vi "Dashboard Main.vi"() -> ()   [LabVIEW 2016]
uses:
  <vilib>/Utility/miscctls.llb/LVRectTypeDef.ctl
  <vilib>/Utility/miscctls.llb/LVPointTypeDef.ctl
  System.Speech
  <vilib>/Rock Robotics/Network Tables/NT Write Number.vi
  <vilib>/Rock Robotics/Network Tables/NT Write Boolean.vi
  <vilib>/Rock Robotics/Network Tables/NT Read Number.vi
  <vilib>/Rock Robotics/Network Tables/NT Read Boolean.vi
  <vilib>/sound2/lvsound2.llb/Sound Output Write (DBL).vi
  Downloads/Beachbot2016Dash-master (1)/Beachbot2016Dash-master/Custom/BB_AutonomousSelector.lvlib
  <vilib>/vision/NI_Vision_Development_Module.lvlib
panel:
  out "Mask 2":T1(plugin-control)
  out "Mask":T1(plugin-control)
  out "Camera Image 2":T1(plugin-control)
  in  "TCP":refnum<k5>
  out "Robot IP":string
  in  "Dashboard Tab":T2(tab)
  out "Gear":u32(colorbox)
  out "NT Connection":bool
  out "Mode":T3(ring)=enum."Auto Disabled"
  out "Shooter RPM":dbl(knob) scale=0.0..3400.0
  out "Air Pressure":dbl(knob) scale=0.0..130.0
  out "Boiler Angle":dbl
  out "Boiler Distance":dbl
  out "In Range":bool=TRUE
  in  "Oscillate":bool=TRUE
  in  "Auto Program":u16(ring) items=["Right Boiler -R- Gear & Shoot", "Right Boiler -L- Gear & Hopper", "Right Boiler 40 Ball v2", "Right Boiler -C- Gear, Shoot & CATCH", "Left Boiler 40 Ball", "Do Nothing", "Right Boiler -C- Gear & Shoot", "Right Boiler -R- Gear Vision & Shoot", "Right Boiler -L- Gear & CATCH", "Left Boiler -C- Gear & Shoot", "Right Boiler 40 Ball", "Left Boiler -L- Gear & Shoot", "Right Boiler -L- Gear & SPRINT"]
  in  "AutoDelay":dbl
  out "MatchTime":i32
  in  "Airship Cam":bool
  in  "Driver Cam":bool
  in  "Shooter Cam":T4={"Hue"={126.19617640889274, 181.21165574429517}, "Sat"={179.10714285714286, 255.0}, "Val"={75.89285714285715, 179.10714285714286}} {"Hue" scale=0.0..255.0 scale format="%#_3g"}
  in  "Driver Cam":T4={"Hue"={104.14999988007006, 130.81818389892578}, "Sat"={157.85714285714286, 255.0}, "Val"={40.53571428571429, 212.5}} {"Hue" scale=0.0..255.0 scale format="%#_3g"}
  out "Tree":string(tree)
  out "Camera Image":T1(plugin-control)
  out "Background":bool
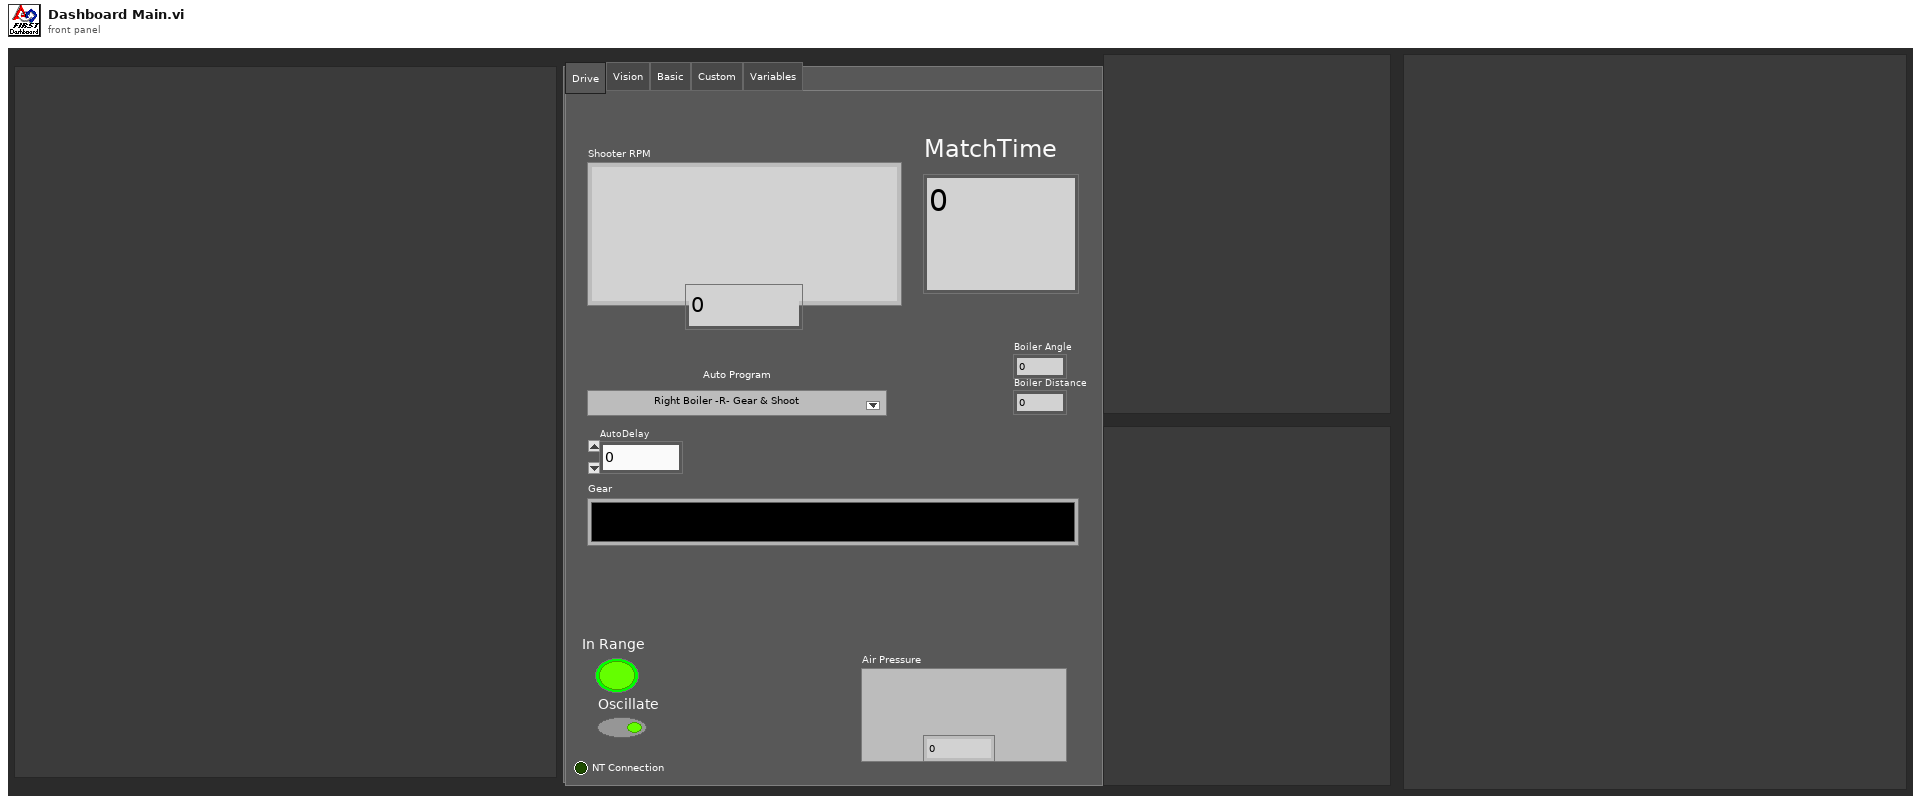
[diagram p1: front panel]
types:
  T1 = typedef "IMAQ Image.ctl" = refnum<image>
  T2 = enum32{"Drive", "Vision", "Basic", "Custom", "Variables"}
  T3 = enum8{"Tele-Op Disabled", "Tele-Op Enabled", "Auto Disabled", "Auto Enabled", "Test Disabled", "Test Enabled", "Disconnected", "No Code", "E-Stop"}
  T4 = cluster{"Hue":cluster{dbl, dbl}, "Sat":cluster{dbl, dbl}, "Val":cluster{dbl, dbl}}
  T5 = typedef "Image Type" = u32
  T6 = typedef "LVPointTypeDef.ctl" = cluster{"Horizontal":i16, "Vertical":i16}
  T7 = typedef "LVRectTypeDef.ctl" = cluster{"Left":i16, "Top":i16, "Right":i16, "Bottom":i16}
  T8 = enum32{"Drive", "Basic", "Custom", "Test", "Checklist", "Variables"}
  T9 = cluster{"Shift":bool, "Ctrl":bool, "Alt":bool, "Cmd":bool, "Opt":bool}
  T10 = cluster{"Error Strings":string, "Disable Counts":cluster{u16, u16}, "Rail Faults":cluster{u16, u16, u16}, "Robot IP":string, "DB Mode":u8, "Event Info":cluster{"Name":string, "Type":u8, "Number":u16, "Replay":u8}}
  T11 = cluster{"Storage":cluster{"Disk Free":u64, "RAM Block":u32, "RAM free":u32}, "CPU Utilization":cluster{"CPU % ISR":sgl, "CPU % Time Crit":sgl, "CPU % Timed Str":sgl, "CPU % High":sgl, "CPU % Above":sgl, "CPU % Normal":sgl, "CPU % Low":sgl}, "CAN":cluster{"% Bus Utilization":sgl, "Bus Off Cnt":u32, "TX_FIFO Full Cnt":u32, "Receive Error Cnt":u8, "Transmit Error Cnt":u8}, "HID":cluster{"HID Outputs":u32, "Rumble Low":u16, "Rumble High":u16}[]}
  T12 = cluster{"Status bits":cluster{"Test Mode":bool, "Autonomous":bool, "Enabled":bool, "Code Start":bool, "Brownout":bool, "Reserved 2":bool, "Reserved 3":bool, "E-Stop":bool}, "Code Trace":cluster{"Disabled":bool, "TeleOp":bool, "Auto":bool, "Test":bool}, "Controller Type":enum16{"unknown", "cRIO", "roboRio"}, "Code?":enum16{"unknown", "noCode", "code"}, "Battery V":dbl}
  T13 = cluster{"Control Bits":cluster{"TestMode":bool, "Autonomous":bool, "Enabled":bool, "FMS Present":bool, bool, bool, bool, "E-Stop":bool}, "Team Station ":u8, "Countdown":sgl, "Joystick Values":cluster{"Axes":dbl[], "Buttons":bool[], "POVs":i16[]}[]}
  T14 = typedef "Sound Output Task ID.ctl" = u32
  T15 = cluster{"Distance (ft)":dbl, "Score":dbl, "Normalized":cluster{"Center":cluster{dbl, dbl}, "Rectangle":cluster{"Numeric":dbl, "Numeric 2":dbl, "Numeric 3":dbl, "Numeric 5":dbl}}, "Pixels":cluster{"Center":cluster{dbl, dbl}, "Rectangle":cluster{"Numeric":dbl, "Numeric 2":dbl, "Numeric 3":dbl, "Numeric 5":dbl}}}
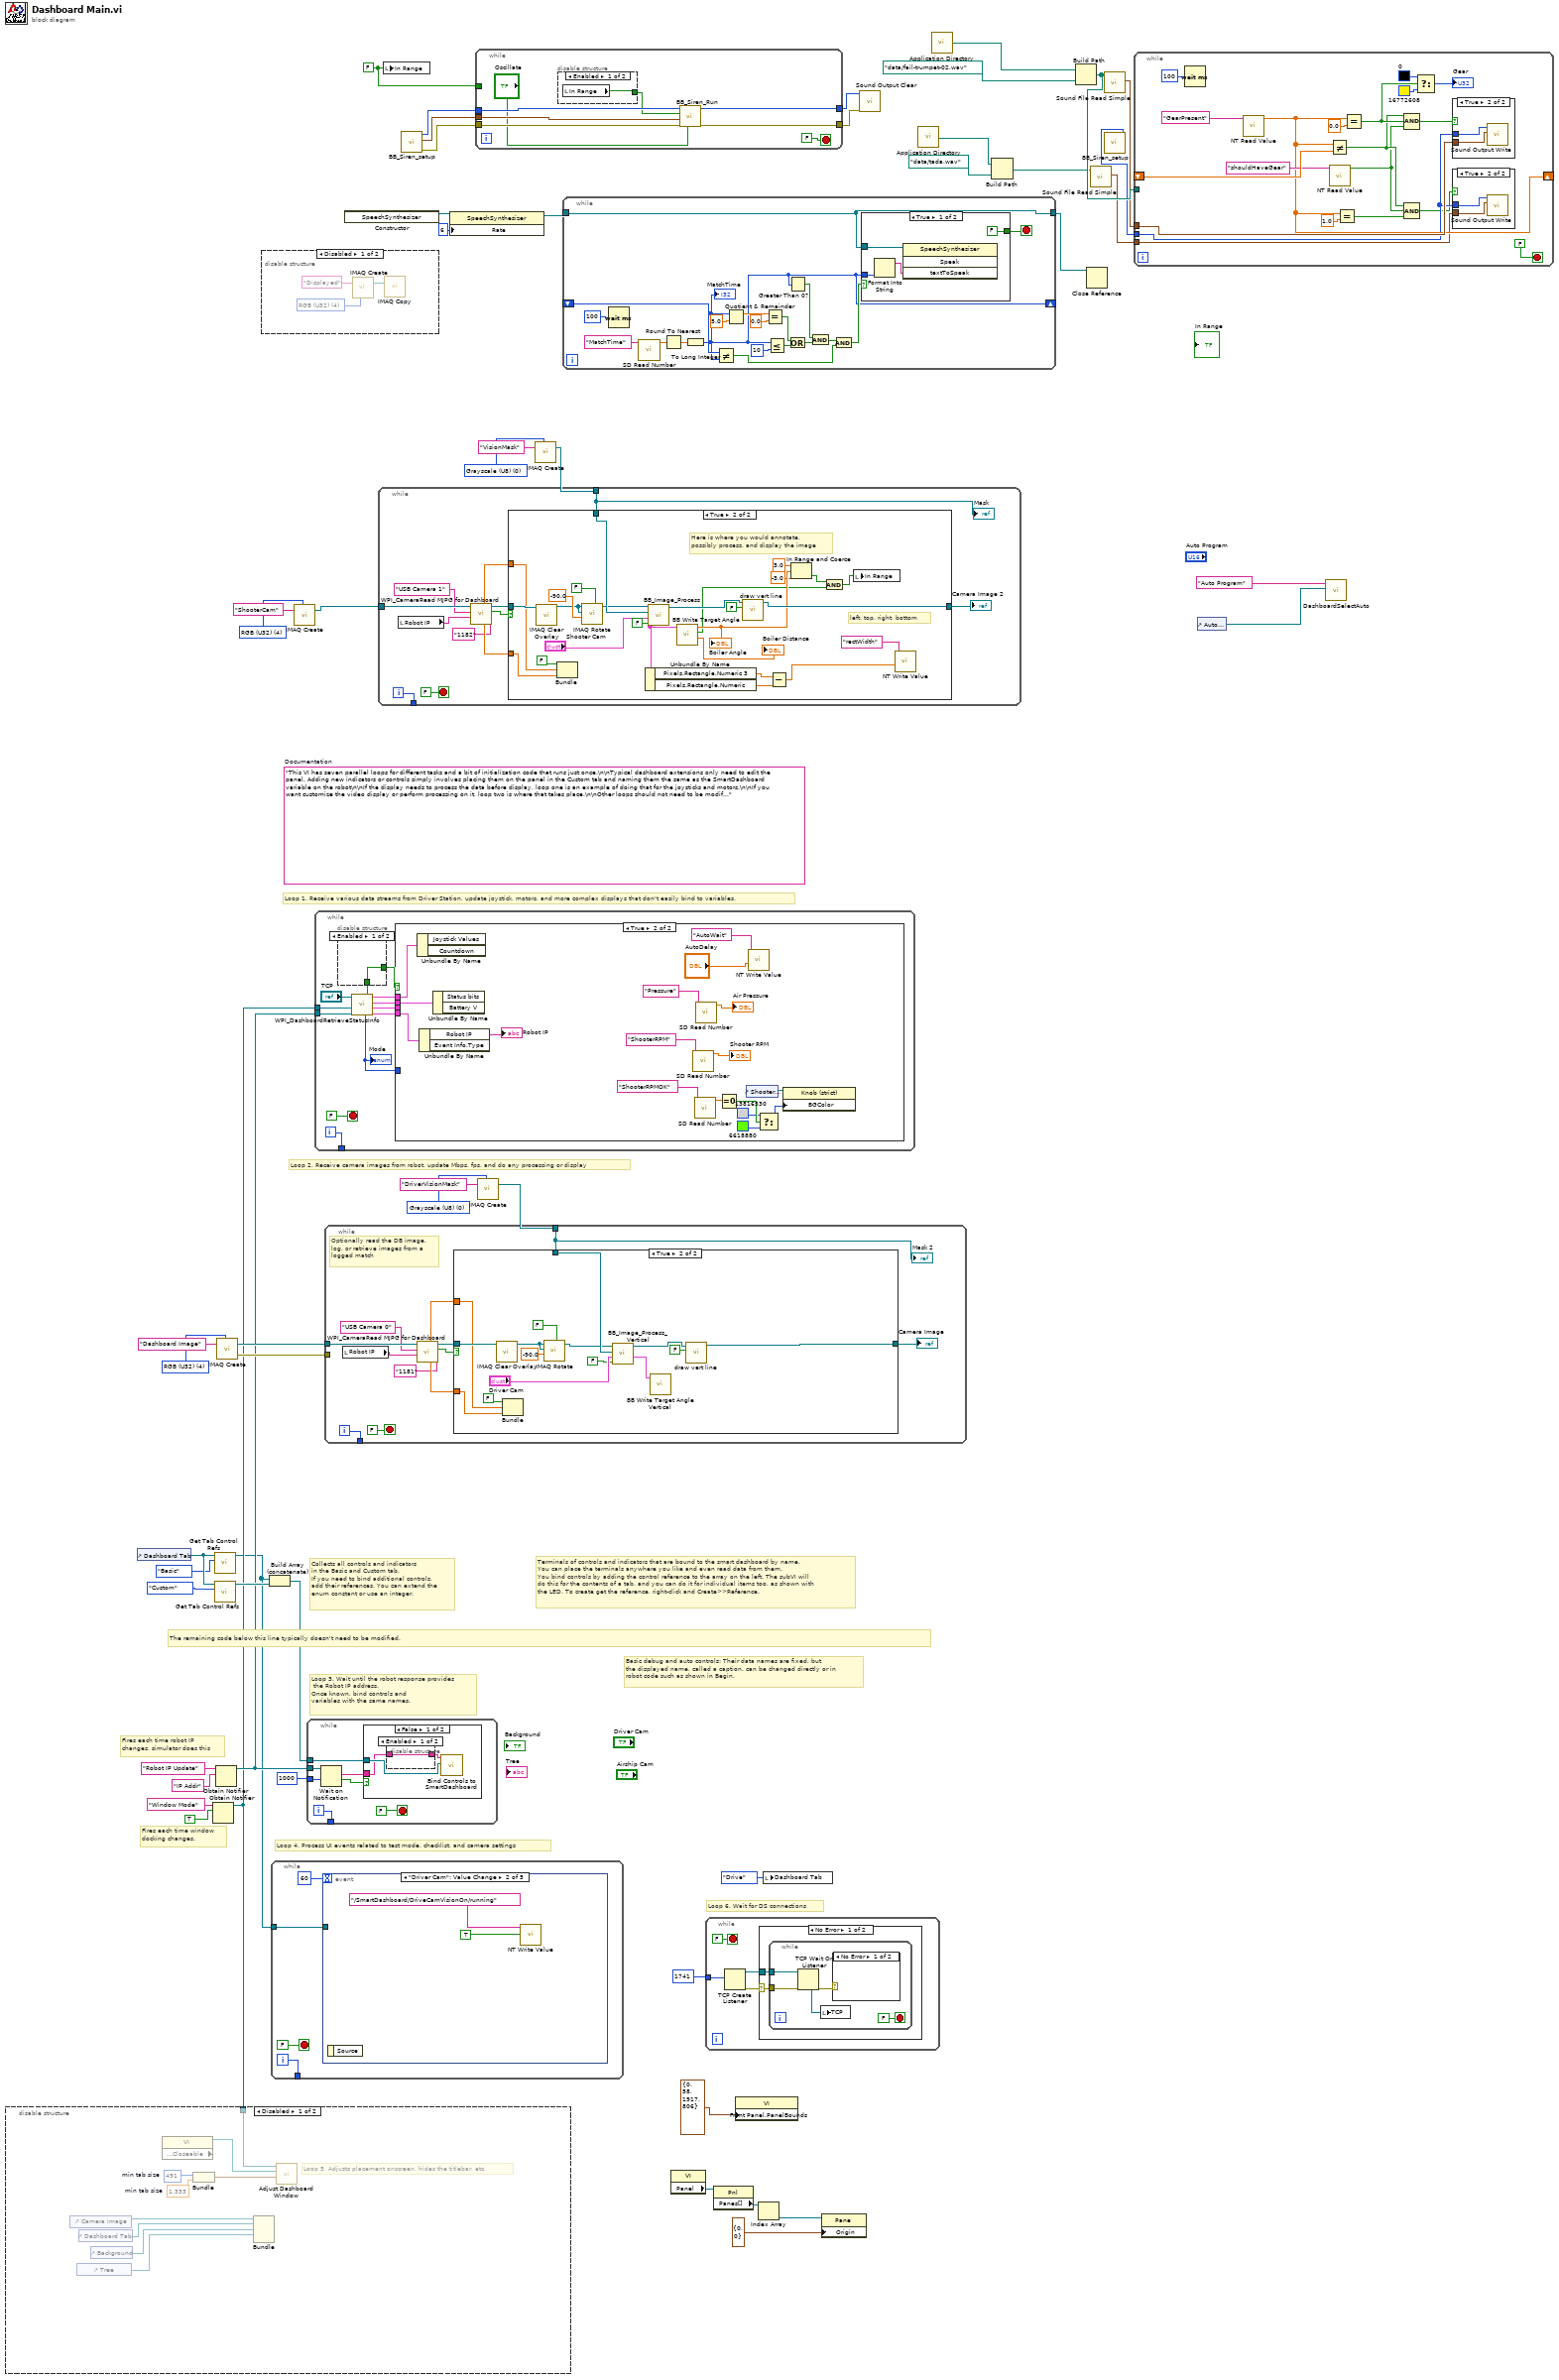
[diagram p0: block diagram]
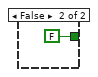
[diagram p2: hidden frame]
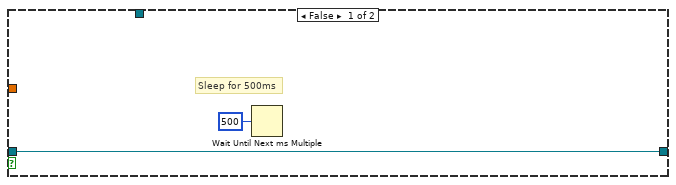
[diagram p5: hidden frame]
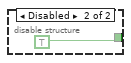
[diagram p6: hidden frame]
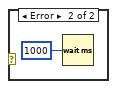
[diagram p9: hidden frame]
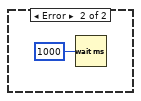
[diagram p10: hidden frame]
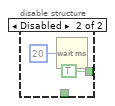
[diagram p11: hidden frame]
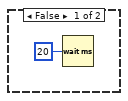
[diagram p12: hidden frame]
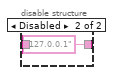
[diagram p13: hidden frame]
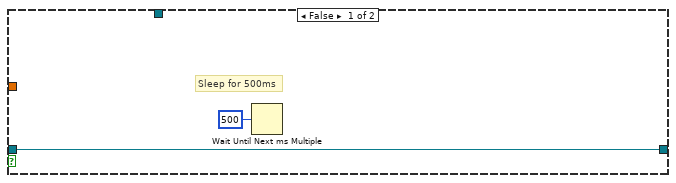
[diagram p15: hidden frame]
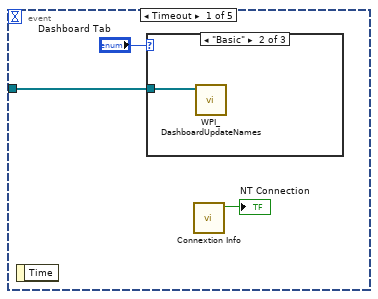
[diagram p16: hidden frame]
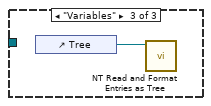
[diagram p18: hidden frame]
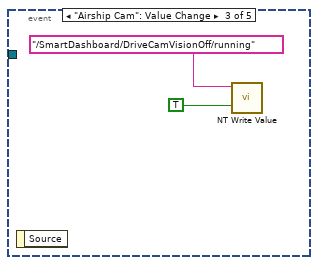
[diagram p19: hidden frame]
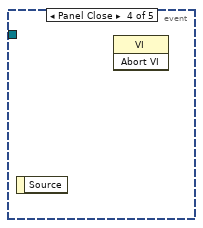
[diagram p20: hidden frame]
diagram:
  w18 = T5 0 items=["Grayscale (U8)", "Grayscale (I16)", "Grayscale (SGL)", "Complex (CSG)", "RGB (U32)", "HSL (U32)", "RGB (U64)"] ("Image Type")
  w21 = T5 4 items=["Grayscale (U8)", "Grayscale (I16)", "Grayscale (SGL)", "Complex (CSG)", "RGB (U32)", "HSL (U32)", "RGB (U64)"] ("Image Type")
  w24 = FALSE ("In Range")
  w30 = T5 0 items=["Grayscale (U8)", "Grayscale (I16)", "Grayscale (SGL)", "Complex (CSG)", "RGB (U32)", "HSL (U32)", "RGB (U64)"] ("Image Type")
  (unwired) "This VI has seven parallel loops for different tasks and a bit of initialization code that runs just once.\n\nTypical dashboard extensions only need to edit the panel. Adding new indicators or controls simply involves placing them on the panel in the Custom tab and naming them the same as the SmartDashboard variable on the robot\n\nIf the display needs to process the data before display, loop one is an example of doing that for the joysticks and motors.\n\nIf you want customize the video display or perform processing on it, loop two is where that takes place.\n\nOther loops should not need to be modified. They are pretty standard, and document the task they perform."  # Documentation
  w54 = T5 4 items=["Grayscale (U8)", "Grayscale (I16)", "Grayscale (SGL)", "Complex (CSG)", "RGB (U32)", "HSL (U32)", "RGB (U64)"] ("Image Type")
  # "Loop 6. Wait for DS connections"
  # "Basic debug and auto controls: Their data names are fixed, but\nthe displayed name, called a caption, can be changed directly or in\nrobot code such as shown in Begin."
  # "Fires each time robot IP\nchanges, simulator does this"
  # "Fires each time window\ndocking changes."
  # "Collects all controls and indicators\nin the Basic and Custom tab.\nIf you need to bind additional controls,\nadd their references. You can extend the\nenum constant or use an integer."
  # "The remaining code below this line typically doesn't need to be modified."
  # "Loop 4. Process UI events related to test mode, checklist, and camera settings"
  # "Terminals of controls and indicators that are bound to the smart dashboard by name.\nYou can place the terminals anywhere you like and even read data from them.\nYou bind controls by adding the control reference to the array on the left. The subVI will\ndo this for the contents of a tab, and you can do it for individual items too, as shown with\nthe LED. To create get the reference, right-click and Create>>Reference."
  # "Loop 3. Wait until the robot response provides\n the Robot IP address.\nOnce known, bind controls and\nvariables with the same names."
  # "Loop 1. Receive various data streams from Driver Station, update joystick, motors, and more complex displays that don't easily bind to variables."
  # "Loop 2. Receive camera images from robot, update Mbps, fps, and do any processing or display"
  n1 = control-ref of="Dashboard Tab"() -> (w45:refnum<vi>)
  n2 = Obtain Notifier(name (unnamed)="Window Mode", notification data type=TRUE) -> (notifier out=w39:refnum<notifier>)  [unwired: 2 in, 2 out]
  n3 = disable-structure shown="Disabled" {
    disable-tunnel: w39 -> [w64 _]
    frame Disabled {
      w60 = 491  # min tab size
      w59 = 1.333  # min tab size
      # "Loop 5. Adjusts placement onscreen, hides the titlebar, etc."
      n4 = control-ref of="Camera Image"() -> (w62:refnum<vi>)
      n5 = control-ref of="Tree"() -> (w56:refnum<vi>)
      n6 = control-ref of="Dashboard Tab"() -> (w61:refnum<vi>)
      n7 = control-ref of="Background"() -> (w57:refnum<vi>)
      n8 = property class="VI" props=["Front Panel.Closeable"]() -> (reference out=w63:refnum<vi>)  [unwired: 2 in, 2 out]
      n9 = Bundle("min tab size"=w60, "min tab size"=w59) -> (w58:cluster{"min tab size":i32, "min tab size":dbl})  [unwired: 1 in]
      n10 = Bundle("Camera Image"=w62, "Dashboard Tab"=w61, "Background"=w57, "Tree"=w56) -> (w55)  [unwired: 1 in, 1 out]
      n11 = call "Adjust Dashboard Window.vi"("Size Constraints"=w58, "VI"=w63, "WIn Mode"=w64) -> ()  [unwired: 9 in]
    }
    frame Enabled {
    }
  }
  n12 = call <vilib>:"Get Tab Control Refs.vi"("Page Index"=T8."Basic" ("Dashboard Tab"), "TabControl in"=w45) -> ("ControlsOnPage"=w37:refnum<vi>[])  [unwired: 9 in]
  n13 = call <vilib>:"Get Tab Control Refs.vi"("Page Index"=T8."Custom" ("Dashboard Tab"), "TabControl in"=w45) -> ("ControlsOnPage"=w44:refnum<vi>[])  [unwired: 9 in]
  n14 = Obtain Notifier(name (unnamed)="Robot IP Update", notification data type="IP Addr" ("name (unnamed)")) -> (notifier out=w40:refnum<notifier>)  [unwired: 2 in, 2 out]
  n15 = call "IMAQ Create"("Image Name"="Dashboard Image", "Image Type"=w54) -> ("New Image"=w52:T1, "error out"=w51:errorcluster)  [unwired: 2 in, 1 out]
  n16 = disable-structure shown="Disabled" {
    frame Disabled {
      w66 = T5 4 items=["Grayscale (U8)", "Grayscale (I16)", "Grayscale (SGL)", "Complex (CSG)", "RGB (U32)", "HSL (U32)", "RGB (U64)"] ("Image Type")
      n17 = call "IMAQ Create"("Image Name"="Displayed", "Image Type"=w66) -> ("New Image"=w65:T1)  [unwired: 2 in, 2 out]
      n18 = call "IMAQ Copy"("Image Src"=w65) -> ()  [unwired: 5 in, 2 out]
    }
    frame Enabled {
    }
  }
  n19 = Build Array (concatenate)(w37, w44) -> (w43:refnum<vi>[])
  n20 = while {
    tunnel: [w69] -> _
    tunnel: w37 -> [w68]
    i -> [w69]
    stop <- FALSE stop-if-true
    n21 = event shown="[1] \"Driver Cam\": Value Change" {
      selector: _ -> [_ _ _ _ _]
      dyn-events: _ -> [_ _ _ _ _]
      timeout: u32 60 ("milliseconds to wait") -> [_ _ _ _ _]
      tunnel: w68 -> [w72 _ _ _ _]
      event Timeout {
        n22 = event-data() -> ()  [unwired: 1 in, 1 out]
        n23 = case shown="\"Basic\"" "Dashboard Tab" {
          tunnel: w72 -> [_ w75 _]
          frame "Custom", Default {
          }
          frame "Basic" {
            n24 = call <vilib>:"WPI_DashboardUpdateNames.vi"("Controls on Tab"=w75) -> ()  [unwired: 11 in]
          }
          frame "Variables" {
            n25 = control-ref of="Tree"() -> (w76:refnum<vi>)
            n26 = call <vilib>:"NT Read and Format Entries as Tree.vi"("Tree Refnum"=w76) -> ()  [unwired: 9 in, 2 out]
          }
        }
        n27 = call <vilib>:"Connextion Info.vi"() -> ("Connected"=→"NT Connection":bool)  [unwired: 10 in, 1 out]
      }
      event "Driver Cam": Value Change {
        n28 = event-data() -> ()  [unwired: 1 in, 1 out]
        n29 = call-poly <vilib>:"NT Write Value.vi"("Boolean"=TRUE, "Name"="/SmartDashboard/DriveCamVisionOn/running") -> ()  [unwired: 9 in, 1 out]
      }
      event "Airship Cam": Value Change {
        n30 = event-data() -> ()  [unwired: 1 in, 1 out]
        n31 = call-poly <vilib>:"NT Write Value.vi"("Boolean"=TRUE, "Name"="/SmartDashboard/DriveCamVisionOff/running") -> ()  [unwired: 9 in, 1 out]
      }
      event Panel Close {
        n32 = event-data() -> ()  [unwired: 1 in, 1 out]
        n33 = invoke class="VI" method="Abort VI"() -> ()  [unwired: 3 in, 3 out]
      }
      event "Tree": Double Click {
        # "Update variable's persistence setting"
        n34 = event-data() -> ("PlatMods"=w84:T9, "Tag"=w83:string)  [unwired: 1 in]
        n35 = Unbundle(w84) -> ("Shift"=w82:bool)  [unwired: 4 out]
        n36 = Not(x=w82) -> (.not. x?=w81:bool)
        n37 = call <vilib>:"NT Update Persistence.vi"("Persistence"=w81, "Name"=w83) -> ()  [unwired: 9 in, 1 out]
      }
    }
  }
  n38 = call "IMAQ Create"("Image Name"="ShooterCam", "Image Type"=w21) -> ("New Image"=w19:T1)  [unwired: 2 in, 2 out]
  n39 = while {
    tunnel: w43 -> [w91]
    tunnel: w40 -> [w89]
    tunnel: [w87] -> _
    tunnel: u32 1000 ("milliseconds to wait") -> [w86]
    i -> [w87]
    stop <- FALSE stop-if-true
    n40 = Wait on Notification(notifier=w89, timeout in ms (-1)=w86) -> (notification=w88:string, timed out?=w85:bool)  [unwired: 2 in, 2 out]
    n41 = case shown="False" w85 {
      tunnel: w91 -> [w94 _]
      tunnel: w88 -> [w93 _]
      frame False {
        n42 = disable-structure shown="Enabled" {
          disable-tunnel: w93 -> [w95 _]
          disable-tunnel: [w95 "127.0.0.1" ("name (unnamed)")] -> w92
          frame Enabled {
          }
          frame Disabled {
          }
        }
        n43 = call <vilib>:"Bind Controls to SmartDashboard.vi"("Bound Control Refs"=w94, "Server IP Address"=w92) -> ()  [unwired: 10 in]
      }
      frame True {
      }
    }
  }
  n44 = while {
    tunnel: [w107] -> _
    tunnel: w40 -> [w102]
    tunnel: w39 -> [w99]
    i -> [w107]
    stop <- FALSE stop-if-true
    n45 = call <vilib>:"WPI_DashboardRetrieveStatusInfo.vi"("Binding Refnum"=w102, "Window Mode Notifier"=w99, "TCP Cnx"="TCP") -> ("Power and Errors"=w103:T10, "Robot Metrics"=w105:T11, "Status Info"=w106:T12, "Control Info"=w104:T13, "Robot Mode"=w101:T3, "Process?"=w98:bool)  [unwired: 3 in]
    "Mode" <- w101
    n46 = disable-structure shown="Enabled" {
      disable-tunnel: [w109 TRUE ("Process?")] -> w97
      disable-tunnel: w98 -> [w109 _]
      frame Enabled {
      }
      frame Disabled {
        n47 = Wait (ms)(milliseconds to wait=u32 20) -> ()  [unwired: 1 out]
      }
    }
    n48 = case shown="True" w97 {
      tunnel: w106 -> [_ w129]
      tunnel: w105 -> [_ _]
      tunnel: w104 -> [_ w128]
      tunnel: w103 -> [_ w127]
      tunnel: w101 -> [_ _]
      frame False {
        n49 = Wait (ms)(milliseconds to wait=u32 20) -> ()  [unwired: 1 out]
      }
      frame True {
        n50 = Unbundle By Name(w128) -> ()  [unwired: 2 out]
        n51 = Unbundle By Name(w127) -> ("Robot IP"=→"Robot IP":string)  [unwired: 1 out]
        n52 = Unbundle By Name(w129) -> ()  [unwired: 2 out]
        n53 = call <vilib>:"SD Read Number.vi"("Name"="ShooterRPM") -> ("Numeric"=→"Shooter RPM":dbl)  [unwired: 8 in, 2 out]
        n54 = call <vilib>:"SD Read Number.vi"("Name"="ShooterRPMOK") -> ("Numeric"=w119:dbl)  [unwired: 8 in, 2 out]
        n55 = call <vilib>:"SD Read Number.vi"("Name"="Pressure") -> ("Numeric"=→"Air Pressure":dbl)  [unwired: 8 in, 2 out]
        n56 = Equal To 0?(x=w119) -> (x = 0?=w118:bool)
        n57 = control-ref of="Shooter RPM"() -> (w120:refnum<vi>)
        n58 = call-poly <vilib>:"NT Write Value.vi"("Numeric"="AutoDelay", "Name"="AutoWait") -> ()  [unwired: 9 in, 1 out]
        n59 = Select(t=u32 13816530, s=w118, f=u32 6618880) -> (s? t:f=w117:u32)
        n60 = property class="Knob (strict)"(reference=w120, "BGColor"=w117) -> ()  [unwired: 1 in, 2 out]
      }
    }
  }
  n61 = constructor class="SpeechSynthesizer"() -> (reference out=w3:refnum<k24>)  [unwired: 3 in, 2 out]
  n62 = local write "In Range"(w24) -> ()
  n63 = call "BB_Siren_setup.vi"() -> ("error out"=w28:errorcluster, "Sampling Info"=w27:cluster{"Fs":dbl, "#s":dbl}, "task ID"=w15:T14)  [unwired: 9 in]
  n64 = property class="SpeechSynthesizer"(reference=w3, "Rate"=6) -> (reference out=w2:refnum<k24>)  [unwired: 1 in, 1 out]
  n65 = while {
    tunnel: w15 -> [w136]
    tunnel: w28 -> [w135]
    tunnel: w27 -> [w134]
    tunnel: [w133] -> w26
    tunnel: [w132] -> w25
    tunnel: w24 -> [_]
    stop <- FALSE stop-if-true
    n66 = disable-structure shown="Enabled" {
      disable-tunnel: [w138 TRUE ("Active")] -> w130
      frame Enabled {
        n67 = local read "In Range"() -> (w138:bool)
      }
      frame Disabled {
      }
    }
    n68 = call "BB_Siren_Run.vi"("Oscillate"="Oscillate", "Error In"=w135, "sampling info"=w134, "Active"=w130, "Task ID In"=w136) -> ("error out"=w133:errorcluster, "task ID out"=w132:T14)  [unwired: 5 in]
  }
  n69 = call "IMAQ Create"("Image Name"="DriverVisionMask", "Image Type"=w30) -> ("New Image"=w9:T1)  [unwired: 2 in, 2 out]
  n70 = while {
    tunnel: w52 -> [w149]
    tunnel: w51 -> [_]
    tunnel: [w150] -> _
    tunnel: w9 -> [w140]
    i -> [w150]
    stop <- FALSE stop-if-true
    # "Optionally read the DB image,\nlog, or retrieve images from a\nlogged match"
    n71 = local read "Robot IP"() -> (w146:string)
    n72 = call "WPI_CameraRead MJPG for Dashboard.vi"("Port"="1181", "Robot IP"=w146, "Camera Name"="USB Camera 0" ("Robot IP"), "Refnum in"=w149) -> ("Active"=w148:bool, "Refnum out"=w141:T1, "FPS"=w147:dbl, "Bandwidth (Mbps)"=w145:dbl)  [unwired: 4 in]
    n73 = case shown="True" w148 {
      tunnel: w141 -> [w152 w168]
      tunnel: w145 -> [_ w166]
      tunnel: w147 -> [_ w167]
      tunnel: [w152 w164] -> w143
      tunnel: w140 -> [_ w162]
      frame False {
        # "Sleep for 500ms"
        n74 = Wait Until Next ms Multiple(millisecond multiple=u32 500) -> ()  [unwired: 1 out]
      }
      frame True {
        n75 = call "IMAQ Clear Overlay"("Image"=w168) -> ("Image Out"=w156:T1)  [unwired: 2 in, 8 out]
        n76 = Bundle(FALSE, "Bandwidth (Mbps)"=w166, "FPS"=w167) -> ()  [unwired: 1 in, 1 out]
        n77 = call "IMAQ Rotate"("Maintain Size"=FALSE, "Angle (degrees)"=sgl -90.0, "Image Dst"=w156, "Image Src"=w156) -> ("Image Dst Out"=w158:T1)  [unwired: 6 in, 1 out]
        n78 = call "BB_Image_Process_Vertical.vi"("Use Calibration"=FALSE, "Color Controls"="Driver Cam", "Mask"=w162, "Input Image"=w158) -> ("Results"=w155:T15, "Original Image"=w161:T1)  [unwired: 5 in, 1 out]
        n79 = call "BB Write Target Angle Vertical.vi"("Results"=w155) -> ()  [unwired: 8 in, 3 out]
        n80 = call "draw vert line.vi"("InRange"=FALSE, "Refnum in"=w161) -> ("Refnum out"=w164:T1)  [unwired: 9 in]
      }
    }
    "Camera Image" <- w143
    "Mask 2" <- w140
  }
  n81 = call "IMAQ Create"("Image Name"="VisionMask", "Image Type"=w18) -> ("New Image"=w10:T1)  [unwired: 2 in, 2 out]
  n82 = while {
    tunnel: w19 -> [w178]
    tunnel: [w179] -> _
    tunnel: w10 -> [w169]
    i -> [w179]
    stop <- FALSE stop-if-true
    n83 = local read "Robot IP"() -> (w171:string)
    n84 = call "WPI_CameraRead MJPG for Dashboard.vi"("Port"="1182", "Robot IP"=w171, "Camera Name"="USB Camera 1" ("Robot IP"), "Refnum in"=w178) -> ("Active"=w176:bool, "Refnum out"=w177:T1, "FPS"=w175:dbl, "Bandwidth (Mbps)"=w174:dbl)  [unwired: 4 in]
    n85 = case shown="True" w176 {
      tunnel: w177 -> [w181 w208]
      tunnel: w174 -> [_ w206]
      tunnel: w175 -> [_ w207]
      tunnel: [w181 w200] -> w173
      tunnel: w169 -> [_ w204]
      frame False {
        # "Sleep for 500ms"
        n86 = Wait Until Next ms Multiple(millisecond multiple=u32 500) -> ()  [unwired: 1 out]
      }
      frame True {
        # "left, top, right, bottom"
        # "Here is where you would annotate,\npossibly process, and display the image"
        n87 = call "IMAQ Clear Overlay"("Image"=w208) -> ("Image Out"=w195:T1)  [unwired: 2 in, 8 out]
        n88 = Bundle(FALSE, "Bandwidth (Mbps)"=w206, "FPS"=w207) -> ()  [unwired: 1 in, 1 out]
        n89 = call "IMAQ Rotate"("Maintain Size"=FALSE, "Angle (degrees)"=sgl -90.0, "Image Dst"=w195, "Image Src"=w195) -> ("Image Dst Out"=w197:T1)  [unwired: 6 in, 1 out]
        n90 = call "BB_Image_Process.vi"("Use Calibration"=FALSE, "Color Controls"="Shooter Cam", "Mask"=w204, "Input Image"=w197) -> ("Results"=w186:T15, "Original Image"=w201:T1)  [unwired: 5 in, 1 out]
        n91 = Unbundle By Name(w186) -> ("Pixels.Rectangle.Numeric 3"=w184:dbl, "Pixels.Rectangle.Numeric"=w185:dbl)
        n92 = call "BB Write Target Angle.vi"("Results"=w186) -> ("TargetDistance"=→"Boiler Distance":dbl, "TargetDetected"=w189:bool, "TargetAngle"=w193:dbl)  [unwired: 8 in]
        "Boiler Angle" <- w193
        n93 = call "draw vert line.vi"("InRange"=FALSE, "Refnum in"=w201) -> ("Refnum out"=w200:T1)  [unwired: 9 in]
        n94 = Subtract(x=w184, y=w185) -> (x-y=w183:dbl)
        n95 = In Range and Coerce(upper limit=3.0, x=w193, lower limit=-3.0) -> (In Range?=w190:bool)  [unwired: 1 out]
        n96 = And(x=w190, y=w189) -> (x .and. y?=w188:bool)
        n97 = local write "In Range"(w188) -> ()
        n98 = call-poly <vilib>:"NT Write Value.vi"("Numeric"=w183, "Name"="rectWidth") -> ()  [unwired: 9 in, 1 out]
      }
    }
    "Camera Image 2" <- w173
    "Mask" <- w169
  }
  n99 = while {
    tunnel: w2 -> [w224]
    shift-right: [w214] -> _
    shift-left: _ -> [w222]
    tunnel: [w224] -> w4
    stop <- w227 stop-if-true
    n100 = Wait (ms)(milliseconds to wait=u32 100) -> ()  [unwired: 1 out]
    n101 = call <vilib>:"SD Read Number.vi"("Name"="MatchTime") -> ("Numeric"=w225:dbl)  [unwired: 8 in, 2 out]
    n102 = Round To Nearest(number=w225) -> (nearest integer value=w215:dbl)
    n103 = To Long Integer(number=w215) -> (32bit integer=w214:i32)
    "MatchTime" <- w214
    n104 = Not Equal?(x=w222, y=w214) -> (x != y?=w220:bool)
    n105 = Quotient & Remainder(x=w214, y=5.0) -> (x-y*floor(x/y)=w217:dbl)  [unwired: 1 out]
    n106 = Equal?(x=w217, y=0.0) -> (x = y?=w211:bool)
    n107 = Less Or Equal?(x=w214, y=10) -> (x <= y?=w210:bool)
    n108 = Greater Than 0?(x=w214) -> (x > 0?=w218:bool)
    n109 = Or(x=w211, y=w210) -> (x .or. y?=w209:bool)
    n110 = And(x=w218, y=w209) -> (x .and. y?=w212:bool)
    n111 = And(x=w212, y=w220) -> (x .and. y?=w219:bool)
    n112 = case shown="True" w219 {
      tunnel: w224 -> [w231 _]
      tunnel: [FALSE FALSE] -> w227
      tunnel: w214 -> [w229 _]
      frame True {
        n113 = Format Into String(w229) -> (resulting string=w228:string)  [unwired: 3 in, 1 out]
        n114 = invoke class="SpeechSynthesizer" method="Speak"(reference=w231, "textToSpeak"=w228) -> ()  [unwired: 2 in, 4 out]
      }
      frame False {
      }
    }
  }
  n115 = property class="VI"() -> ("Panel"=w35:refnum<vi>)  [unwired: 2 in, 2 out]
  n116 = while {
    tunnel: u16 1741 ("timeout ms (25000)") -> [w234]
    stop <- FALSE stop-if-true
    n117 = TCP Create Listener(10:w234) -> (0:w233:errorcluster, 3:w235:refnum<k5>)  [unwired: 4 in, 1 out]
    n118 = case shown="No Error" w233 {
      selector: w233 -> [w237 _]
      tunnel: w235 -> [w238 _]
      frame No Error {
        n119 = while {
          tunnel: w238 -> [w241]
          tunnel: w237 -> [w240]
          stop <- FALSE stop-if-true
          n120 = TCP Wait On Listener(8:w240, 11:w241) -> (0:w242:errorcluster, 4:w243:refnum<k5>)  [unwired: 2 in, 3 out]
          n121 = local write "TCP"(w243) -> ()
          n122 = case shown="No Error" w242 {
            frame No Error {
            }
            frame Error {
              n123 = Wait (ms)(milliseconds to wait=u32 1000) -> ()  [unwired: 1 out]
            }
          }
        }
      }
      frame Error {
        n124 = Wait (ms)(milliseconds to wait=u32 1000) -> ()  [unwired: 1 out]
      }
    }
  }
  n125 = property class="Pnl"(reference=w35) -> ("Panes[]"=w34:refnum<vi>[])  [unwired: 1 in, 2 out]
  n126 = property class="VI"("Front Panel.PanelBounds"=T7 {"Left"=0, "Top"=58, "Right"=1917, "Bottom"=806} ("Front Panel Window:Panel Bounds")) -> ()  [unwired: 2 in, 2 out]
  n127 = Index Array(array=w34) -> (element=w33:refnum<vi>)  [unwired: 1 in]
  n128 = local write "Dashboard Tab"(T2."Drive" ("Dashboard Tab")) -> ()
  n129 = property class="Pane"(reference=w33, "Origin"=T6 {"Horizontal"=0, "Vertical"=0}) -> ()  [unwired: 1 in, 2 out]
  n130 = call <vilib>:"Sound Output Clear.vi"("error in (no error)"=w26, "task ID"=w25) -> ()  [unwired: 9 in, 1 out]
  n131 = call <vilib>:"Application Directory.vi"() -> ("Application Directory"=w8:path)
  n132 = call <vilib>:"Application Directory.vi"() -> ("Application Directory"=w11:path)
  n133 = Build Path(base path=w8, name or relative path=path "data/tada.wav" ("Sound File Path")) -> (appended path=w7:path)
  n134 = Build Path(base path=w11, name or relative path=path "data/fail-trumpet-02.wav" ("Sound File Path")) -> (appended path=w14:path)
  n135 = Close Reference(reference=w4) -> ()  [unwired: 1 in, 1 out]
  n136 = call <vilib>:"Sound File Read Simple.vi"("path"=w7) -> ("data"=w5:waveform(dbl)[])  [unwired: 7 in, 3 out]
  n137 = call <vilib>:"Sound File Read Simple.vi"("path"=w14) -> ("data"=w12:waveform(dbl)[])  [unwired: 7 in, 3 out]
  n138 = call "BB_Siren_setup.vi"() -> ("task ID"=w13:T14)  [unwired: 9 in, 2 out]
  n139 = while {
    tunnel: w14 -> [_]
    tunnel: w13 -> [w248]
    tunnel: w12 -> [w264]
    shift-right: [w252] -> _
    shift-left: _ -> [w263]
    tunnel: w5 -> [w246]
    stop <- FALSE stop-if-true
    n140 = Wait (ms)(milliseconds to wait=u32 100) -> ()  [unwired: 1 out]
    n141 = call-poly <vilib>:"NT Read Value.vi"("Name"="GearPresent") -> ("Numeric"=w252:dbl)  [unwired: 9 in, 1 out]
    n142 = Not Equal?(x=w252, y=w263) -> (x != y?=w250:bool)
    n143 = call-poly <vilib>:"NT Read Value.vi"("Name"="shouldHaveGear") -> ("Boolean"=w249:bool)  [unwired: 9 in, 1 out]
    n144 = Equal?(x=w252, y=1.0) -> (x = y?=w251:bool)
    n145 = Equal?(x=w252, y=0.0) -> (x = y?=w254:bool)
    n146 = Compound Arithmetic op=AND(w250, w254, w249) -> (w259:bool)
    n147 = Compound Arithmetic op=AND(w250, w249, w251) -> (w247:bool)
    n148 = Select(t=u32 0 ("Gear"), s=w254, f=u32 16772608 ("Gear")) -> (s? t:f=→"Gear":u32)
    n149 = case shown="True" w259 {
      tunnel: w248 -> [_ w269]
      tunnel: w264 -> [_ w268]
      frame False {
      }
      frame True {
        n150 = call-poly <vilib>:"Sound Output Write.vi"("data"=w268, "task ID"=w269) -> ()  [unwired: 8 in, 2 out]
      }
    }
    n151 = case shown="True" w247 {
      tunnel: w248 -> [_ w267]
      tunnel: w246 -> [_ w266]
      frame False {
      }
      frame True {
        n152 = call-poly <vilib>:"Sound Output Write.vi"("data"=w266, "task ID"=w267) -> ()  [unwired: 8 in, 2 out]
      }
    }
  }
  n153 = control-ref of="Auto Program"() -> (w23:refnum<vi>)
  n154 = call "DashboardSelectAuto.vi"("Table Prefix"="Auto Program", "Autonomous Mode Ring"=w23) -> ()  [unwired: 9 in]
